vi "FindVISAResource.vi"(7 "error in":errorcluster, 9 "串口配置In":T1={"端口选择"="COM2", "波特率"=57600, "数据位"=8, "奇偶校验"=0, "停止位"=10, "流控"=0} {"流控" items=["None"=0, "XON/XOFF"=1, "RTS/CTS"=2, "DTR/DSR"=4]; "停止位" items=["1.0"=10, "1.5"=15, "2.0"=20]; "奇偶校验" items=["None", "Odd", "Even", "Mark", "Space"]; "数据位" min=5 max=8 step=1}, 10 "USB-SERIAL name":string="USB-SERIAL") -> (0 "error out":errorcluster, 3 "串口配置Out":T1={"端口选择"=" ", "波特率"=115200, "数据位"=8, "奇偶校验"=0, "停止位"=10, "流控"=0} {"流控" items=["None"=0, "XON/XOFF"=1, "RTS/CTS"=2, "DTR/DSR"=4]; "停止位" items=["1.0"=10, "1.5"=15, "2.0"=20]; "奇偶校验" items=["None", "Odd", "Even", "Mark", "Space"]; "数据位" min=5 max=8 step=1})   [LabVIEW 2015]
uses:
  <vilib>/Instr/_visa.llb/VISA Find Search Mode.ctl
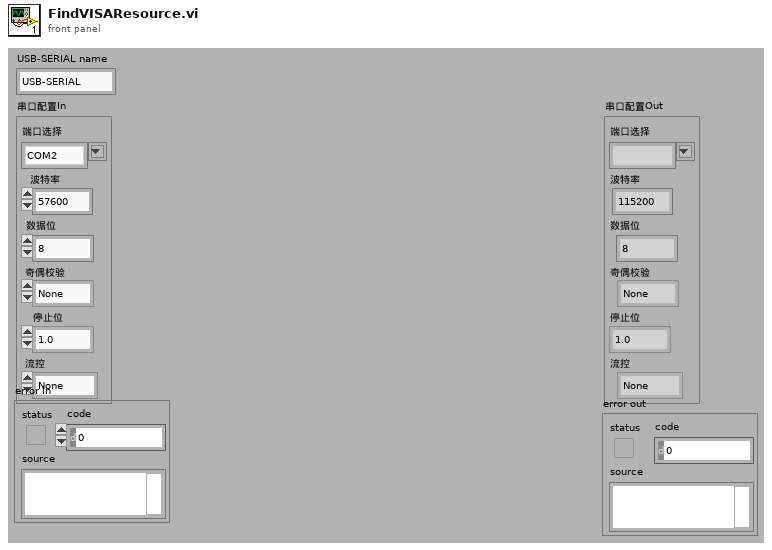
[diagram p1: front panel]
types:
  T1 = cluster{"端口选择":string, "波特率":u32, "数据位":u16, "奇偶校验":u16, "停止位":u16, "流控":u16}
  T2 = typedef "VISA Find Search Mode.ctl" = u32
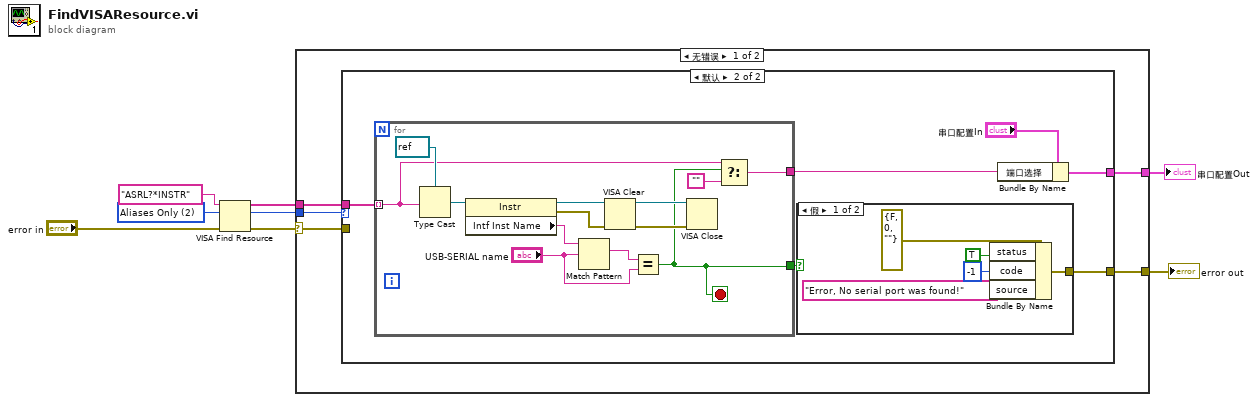
[diagram p0: block diagram]
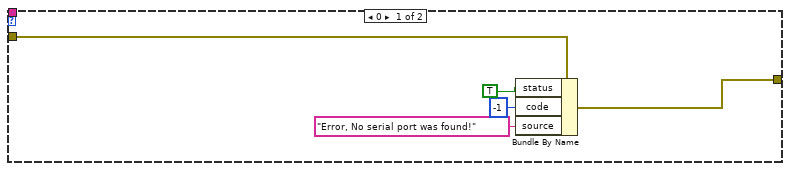
[diagram p2: hidden frame]
diagram:
  w3 = T2 2 items=["Canonical Names Only"=0, "Aliases Only"=2, "Include Matching Aliases"=3, "Include All Aliases"=4] ("Search Mode")
  n1 = VISA Find Resource(8:"error in", 10:w3, 11:"ASRL?*INSTR" ("expression (\"?*\")")) -> (0:w1:errorcluster, 2:w7:u32, 3:w8:string[])
  n2 = case shown="无错误" w1 {
    selector: w1 -> [w9 w43]
    tunnel: w8 -> [w13 _]
    tunnel: w7 -> [w12 _]
    tunnel: [w11 _] -> w6
    tunnel: [w10 w43] -> w4
    frame No Error {
      n3 = case shown="默认" w12 {
        tunnel: w13 -> [_ w24]
        tunnel: [_ w22] -> w11
        tunnel: w9 -> [w18 _]
        tunnel: [w16 w19] -> w10
        frame 0 {
          n4 = Bundle By Name(cluster=w18, "status"=TRUE, "code"=-1, "source"="Error, No serial port was found!") -> (w16:errorcluster)
        }
        frame Default {
          n5 = for {
            tunnel: w24 -> [w37] mode=indexing
            tunnel: [w35] -> w23
            tunnel: [w30] -> w20
            stop <- w30 stop-if-true
            n6 = Type Cast(type=refnum<visa-resource-name> refnum ("reference"), x=w37) -> (*(type *) &x=w41:refnum<visa-resource-name>)
            n7 = property class="Instr"(reference=w41) -> (reference out=w33:refnum<visa-resource-name>, error out=w32:errorcluster, "Intf Inst Name"=w40:string)  [unwired: 1 in]
            n8 = Match Pattern(string=w40, regular expression="USB-SERIAL name") -> (match substring=w39:string)  [unwired: 4 out]
            n9 = VISA Clear(VISA resource name=w33, error in (no error)=w32) -> (VISA resource name out=w34:refnum<visa-resource-name>, error out=w31:errorcluster)
            n10 = Equal?(x=w39, y="USB-SERIAL name") -> (x = y?=w30:bool)
            n11 = VISA Close(VISA resource name=w34, error in (no error)=w31) -> ()  [unwired: 1 out]
            n12 = Select(t=w37, s=w30, f="") -> (s? t:f=w35:string)
          }
          n13 = case shown="假" w20 {
            tunnel: [w26 _] -> w19
            frame False {
              n14 = Bundle By Name(cluster=errorcluster {"status"=FALSE, "code"=0, "source"=""} ("error constant"), "status"=TRUE, "code"=-1, "source"="Error, No serial port was found!") -> (w26:errorcluster)
            }
            frame True {
            }
          }
          n15 = Bundle By Name(cluster="串口配置In", "端口选择"=w23) -> (w22:T1)
        }
      }
    }
    frame Error {
    }
  }
  "串口配置Out" <- w6
  "error out" <- w4
